vi "Measure.vi"(6 "error in (no error)":errorcluster, 9 "Tektronix PA1000 in":refnum<class "Tektronix PA1000.lvclass">) -> (0 "error out":errorcluster, 2 "Array of Measurement":dbl[](array[numeric]), 3 "Tektronix PA1000 out":refnum<class "Tektronix PA1000.lvclass">)   [LabVIEW 2013, in "Universal Power Meter.lvlib" / "Tektronix PA1000.lvlib" / "Tektronix PA1000.lvclass"]
uses:
  Tektronix PA1000.lvclass
  Universal Power Meter class/Universal Power Meter.lvclass
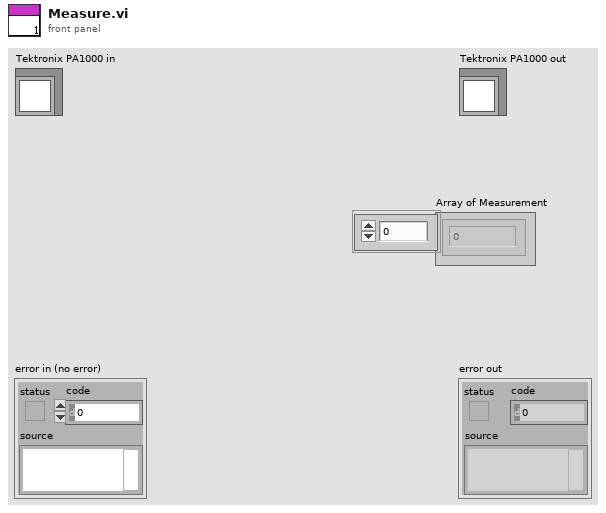
[diagram p1: front panel]
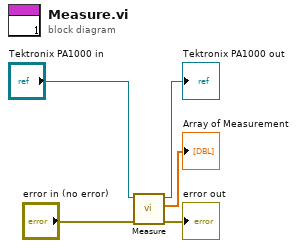
[diagram p0: block diagram]
diagram:
  n1 = call-parent "Measure.vi"("error in (no error)"="error in (no error)", "Universal Power Meter in"="Tektronix PA1000 in") -> ("error out"=→"error out":errorcluster, "Array of Measurement"=→"Array of Measurement":dbl[], "Universal Power Meter out"=→"Tektronix PA1000 out":refnum<class "Tektronix PA1000.lvclass">)  [unwired: 5 in]
